vi "Controls UI.vi"(8 "error in (no error)":errorcluster, 11 "App in":refnum<class "App.lvclass">) -> (0 "error out":errorcluster, 3 "App out":refnum<class "App.lvclass">)   [LabVIEW 2022 SP3, in "VMR-Deck.lvlib" / "App.lvclass"]
uses:
  App.lvclass
  <vilib>/IlluminatedG/IG VoicemeeterRemote API/VoiceMeeterRemote/Direction.ctl
  App.lvclass/App.ctl
  VMR/VMR.lvclass
  <vilib>/IlluminatedG/IG VoicemeeterRemote API/VoiceMeeterRemote/VoiceMeeterRemote.lvlib
panel:
  in  "Speakers":bool
  in  "Mic":bool
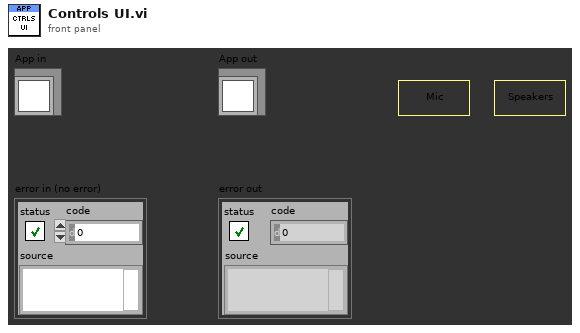
[diagram p1: front panel]
types:
  T1 = typedef "VoiceMeeterRemote.lvlib/Direction.ctl" = enum16{"Input", "Output"}
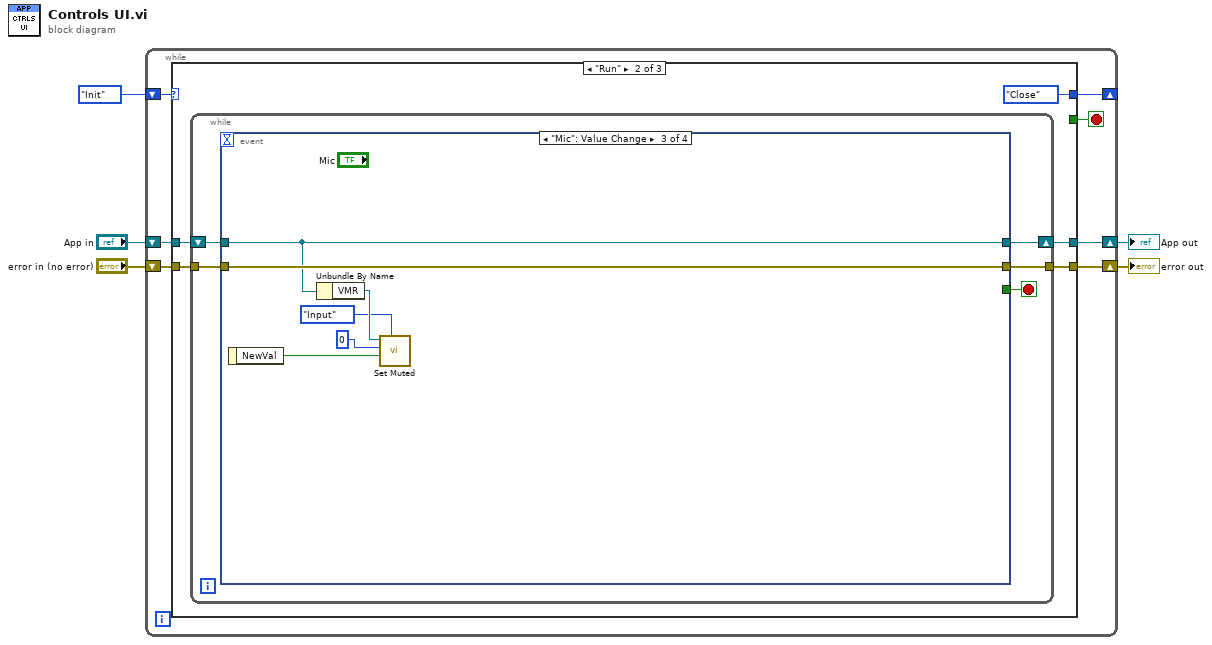
[diagram p0: block diagram]
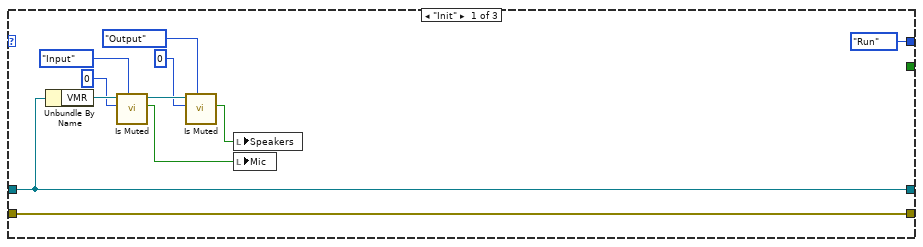
[diagram p2: hidden frame]
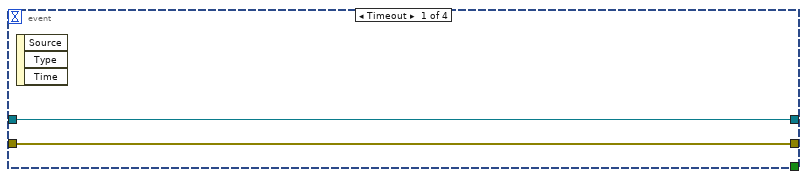
[diagram p3: hidden frame]
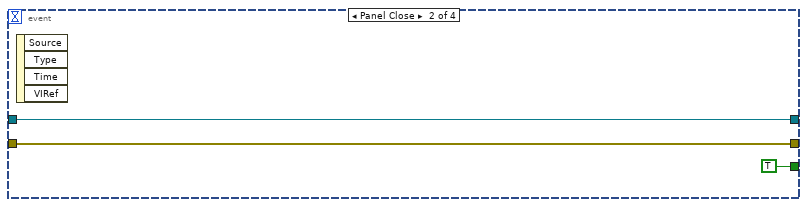
[diagram p4: hidden frame]
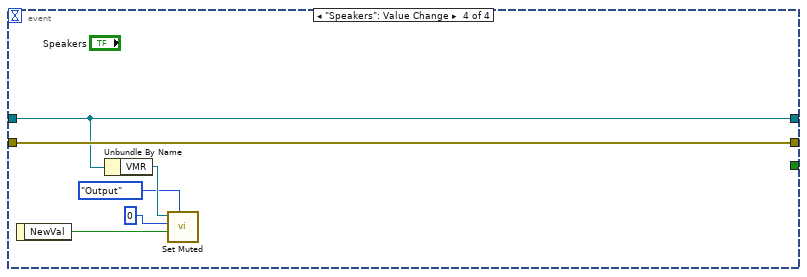
[diagram p5: hidden frame]
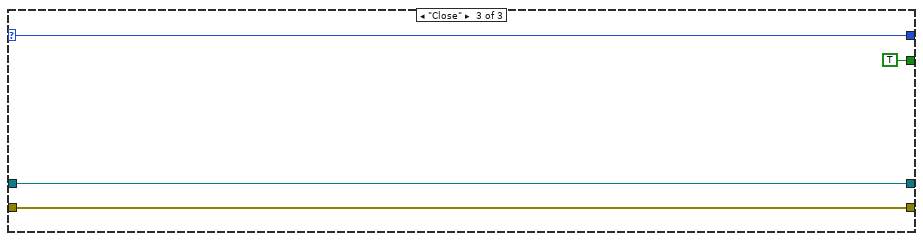
[diagram p6: hidden frame]
diagram:
  n1 = while {
    shift-right: [w11] -> _
    shift-left: enum16{"Init", "Run", "Close"}."Init" -> [w12]
    shift-right: [w6] -> w2
    shift-left: "App in" -> [w9]
    shift-right: [w7] -> w1
    shift-left: "error in (no error)" -> [w8]
    stop <- w10 stop-if-true
    n2 = case shown="\"Run\"" w12 {
      selector: w12 -> [_ _ w54]
      tunnel: [enum16{"Init", "Run", "Close"}."Run" enum16{"Init", "Run", "Close"}."Close" w54] -> w11
      tunnel: [_ _ TRUE] -> w10
      tunnel: w9 -> [w13 w27 w52]
      tunnel: w8 -> [w22 w26 w51]
      tunnel: [w22 w24 w51] -> w7
      tunnel: [w13 w25 w52] -> w6
      frame "Init" {
        n3 = Unbundle By Name(w13) -> ("VMR"=w21:refnum<class "VMR.lvclass">)
        n4 = call "Is Muted.vi"("Direction"=Direction."Input", "Index"=0, "VMR in"=w21) -> ("Muted"=w15:bool, "VMR out"=w18:refnum<class "VMR.lvclass">)  [unwired: 6 in, 1 out]
        n5 = call "Is Muted.vi"("Direction"=Direction."Output", "Index"=0, "VMR in"=w18) -> ("Muted"=w14:bool)  [unwired: 6 in, 2 out]
        n6 = local write "Speakers"(w14) -> ()
        n7 = local write "Mic"(w15) -> ()
      }
      frame "Run" {
        n8 = while {
          shift-right: [w32] -> w25
          shift-left: w27 -> [w33]
          tunnel: w26 -> [w31]
          tunnel: [w30] -> w24
          stop <- w29 stop-if-true
          n9 = event shown="[2] \"Mic\": Value Change" {
            selector: _ -> [_ _ _ _]
            dyn-events: _ -> [_ _ _ _]
            timeout: _ -> [_ _ _ _]
            tunnel: w33 -> [w35 w38 w43 w49]
            tunnel: [w35 w38 w43 w49] -> w32
            tunnel: w31 -> [w34 w37 w44 w50]
            tunnel: [w34 w37 w44 w50] -> w30
            tunnel: [_ TRUE _ _] -> w29
            event Timeout {
              n10 = event-data() -> ()  [unwired: 1 in, 3 out]
            }
            event Panel Close {
              n11 = event-data() -> ()  [unwired: 1 in, 4 out]
            }
            event "Mic": Value Change {
              n12 = event-data() -> ("NewVal"=w41:bool)  [unwired: 1 in]
              n13 = Unbundle By Name(w43) -> ("VMR"=w42:refnum<class "VMR.lvclass">)
              n14 = call "Set Muted.vi"("Direction"=Direction."Input", "Mute"=w41, "Index"=0, "VMR in"=w42) -> ()  [unwired: 6 in, 2 out]
            }
            event "Speakers": Value Change {
              n15 = event-data() -> ("NewVal"=w47:bool)  [unwired: 1 in]
              n16 = Unbundle By Name(w49) -> ("VMR"=w48:refnum<class "VMR.lvclass">)
              n17 = call "Set Muted.vi"("Direction"=Direction."Output", "Mute"=w47, "Index"=0, "VMR in"=w48) -> ()  [unwired: 6 in, 2 out]
            }
          }
        }
      }
      frame "Close" {
      }
    }
  }
  "error out" <- w1
  "App out" <- w2
